vi "Control - Hybrid Engine.vi"() -> ()   [LabVIEW 2013]
uses:
  Control 2.ctl
  <vilib>/DAQmx/write.llb/DAQmx Write (Digital Bool 1Line 1Point).vi
  <vilib>/DAQmx/miscellaneous.llb/DAQmx Fill In Error Info.vi
panel:
  out "OFF":bool
  in  "Servo OFF Com":bool
  in  "Close Command":string="close!"
  in  "Open Command":string="open!"
  in  "Stop Button":bool
  in  "VISA resource name":refnum<visa-resource-name>="COM3"
  out "Servo Off":bool
  out "Servo On":bool
  in  "Serial Settings":T1={"baud rate"=9600, "data bits"=8, "parity"=enum."None", "stop bits"=10, "flow control"=0} {"flow control" items=["None"=0, "XON/XOFF"=1, "RTS/CTS"=2, "DTR/DSR"=4]; "stop bits" items=["1.0"=10, "1.5"=15, "2.0"=20]; "data bits" min=5 max=8 step=1; "baud rate" items=["75"=75, "110"=110, "134"=134, "150"=150, "300"=300, "600"=600, "1200"=1200, "1800"=1800, "2400"=2400, "4800"=4800, "7200"=7200, "9600"=9600, "14400"=14400, "19200"=19200, "28800"=28800, "38400"=38400, "56000"=56000, "57600"=57600, "115200"=115200, "128000"=128000, "230400"=230400]}
  in  "Servo ON Com":bool
  in  "Oxygen Flood":bool
  in  "Ignition":bool
  out "Disconnected":bool
  out "Solenoid \nClosed":bool
  out "Closed":bool
  out "READY":bool
  in  "Fill Line":bool
  out "FILL TANK EMPTYING":bool
  out "Venting":bool
  out "Filling":bool
  in  "Fill Line Vent":bool
  in  "Oxidizer Fill":bool
  # "***************THIS PROGRAM MUST BE RUNNING CONSTANTLY WHEN SOLENOIDS ARE CONNECTED"
  # "Engine Ignition"
  # "Oxidizer Filling"
  # "Manual Control"
  # "Must hold down to be activated"
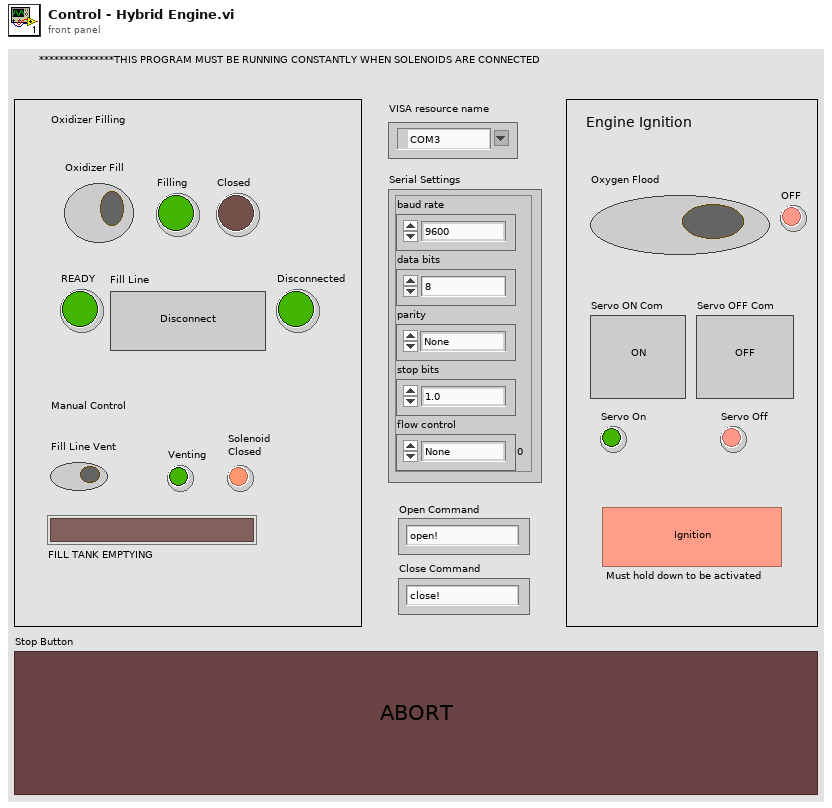
[diagram p1: front panel]
types:
  T1 = typedef "Control 2.ctl" = cluster{"baud rate":u32, "data bits":u16, "parity":enum16{"None", "Odd", "Even", "Mark", "Space"}, "stop bits":u16, "flow control":u16}
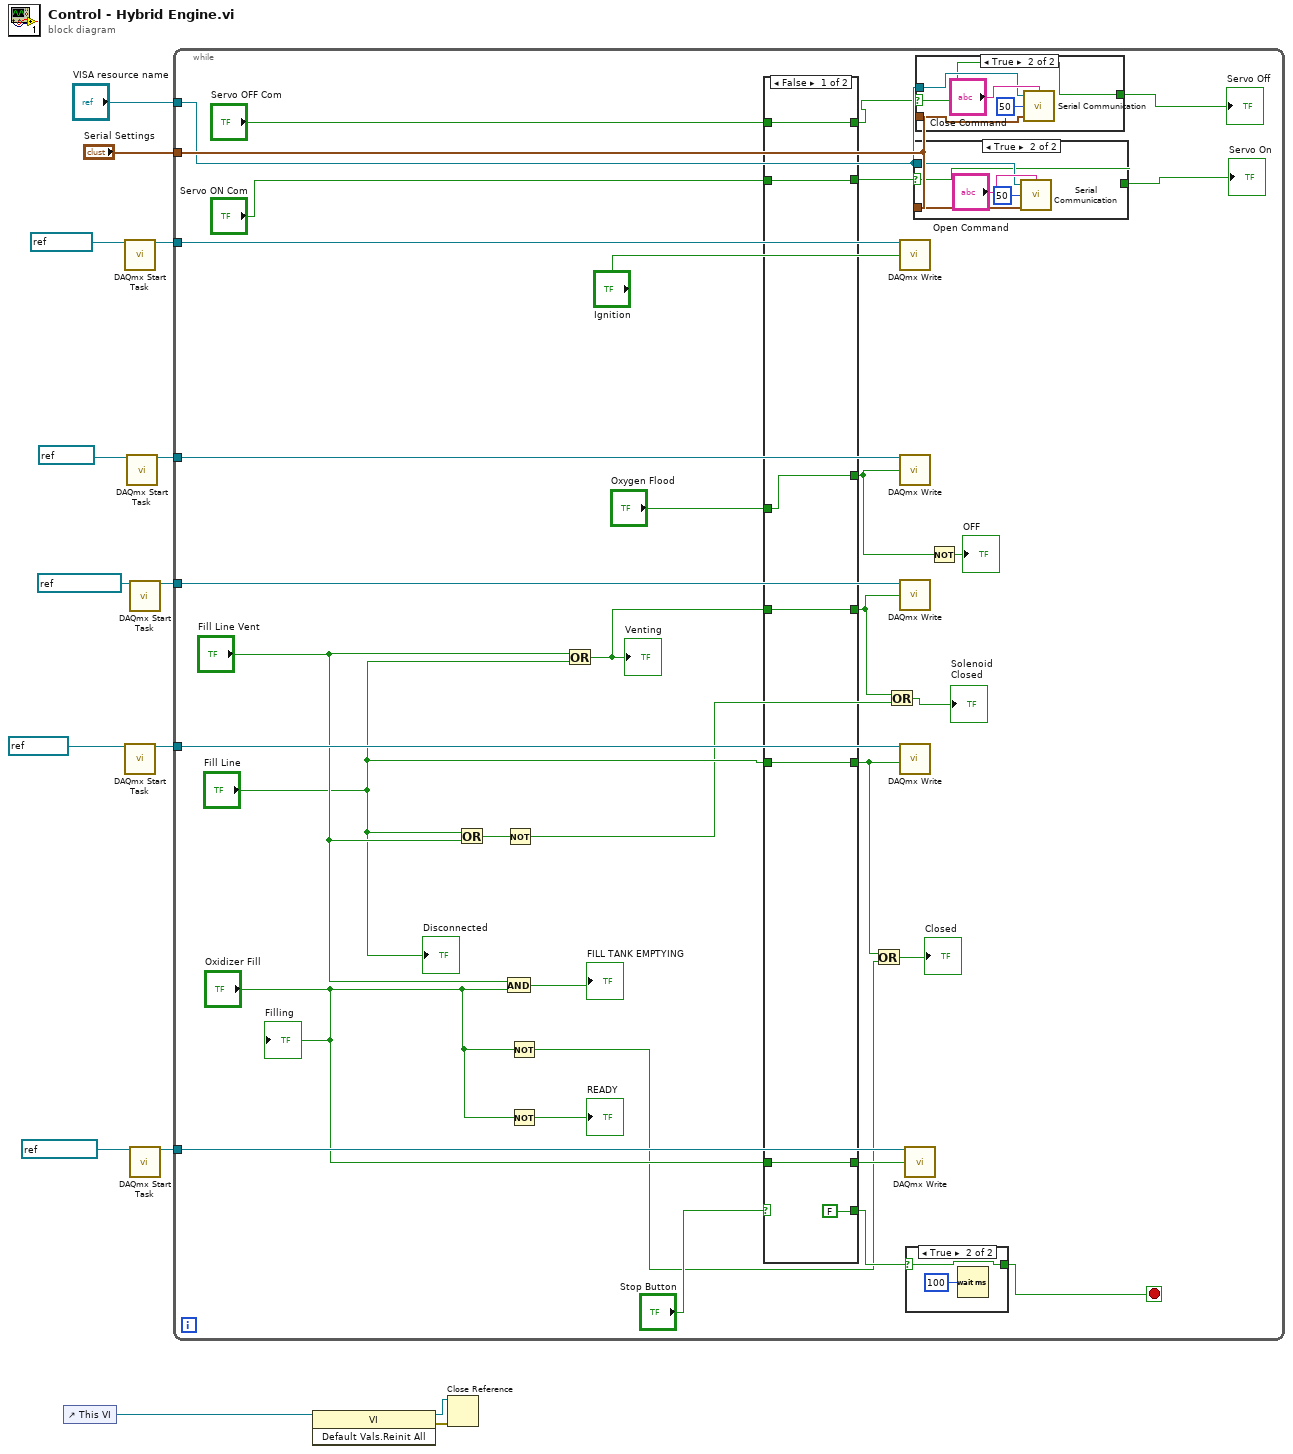
[diagram p0: block diagram]
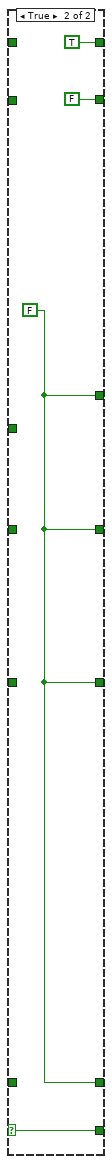
[diagram p3: hidden frame]
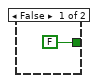
[diagram p4: hidden frame]
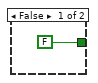
[diagram p5: hidden frame]
diagram:
  n1 = control-ref of="This VI"() -> (w1:refnum<vi>)
  n2 = call <vilib>:"DAQmx Start Task.vi"("task/channels in"=refnum<k21> "Igniter") -> ("task out"=w13:refnum<k21>)  [unwired: 13 in, 1 out]
  n3 = call <vilib>:"DAQmx Start Task.vi"("task/channels in"=refnum<k21> "AUX 1") -> ("task out"=w15:refnum<k21>)  [unwired: 13 in, 1 out]
  n4 = call <vilib>:"DAQmx Start Task.vi"("task/channels in"=refnum<k21> "O2fill") -> ("task out"=w6:refnum<k21>)  [unwired: 13 in, 1 out]
  n5 = call <vilib>:"DAQmx Start Task.vi"("task/channels in"=refnum<k21> "NOS VENT") -> ("task out"=w8:refnum<k21>)  [unwired: 13 in, 1 out]
  n6 = call <vilib>:"DAQmx Start Task.vi"("task/channels in"=refnum<k21> "NOS FILL") -> ("task out"=w14:refnum<k21>)  [unwired: 13 in, 1 out]
  n7 = while {
    tunnel: w15 -> [w49]
    tunnel: w14 -> [w48]
    tunnel: w13 -> [w47]
    tunnel: w8 -> [w46]
    tunnel: w6 -> [w44]
    tunnel: "VISA resource name" -> [w38]
    tunnel: "Serial Settings" -> [w39]
    stop <- w24 stop-if-true
    n8 = Or(x="Fill Line", y="Fill Line Vent") -> (x .or. y?=w42:bool)
    n9 = And(x="Fill Line Vent", y="Oxidizer Fill") -> (x .and. y?=→"FILL TANK EMPTYING":bool)
    n10 = Not(x=w42) -> (.not. x?=w20:bool)
    n11 = Not(x="Oxidizer Fill") -> (.not. x?=w23:bool)
    n12 = Not(x="Oxidizer Fill") -> (.not. x?=→"READY":bool)
    n13 = Or(x="Fill Line Vent", y="Fill Line") -> (x .or. y?=w30:bool)
    "Venting" <- w30
    n14 = case shown="False" "Stop Button" {
      selector: "Stop Button" -> [_ w60]
      tunnel: [w59 FALSE] -> w35
      tunnel: "Servo ON Com" -> [w59 _]
      tunnel: "Servo OFF Com" -> [w58 _]
      tunnel: [w58 TRUE] -> w32
      tunnel: "Oxygen Flood" -> [w57 _]
      tunnel: [w57 w63] -> w16
      tunnel: w30 -> [w56 _]
      tunnel: [w56 w63] -> w19
      tunnel: "Fill Line" -> [w55 _]
      tunnel: [w55 w63] -> w22
      tunnel: "Oxidizer Fill" -> [w54 _]
      tunnel: [w54 w63] -> w27
      tunnel: [FALSE w60] -> w25
      frame False {
      }
      frame True {
        w63 = FALSE
      }
    }
    n15 = Or(x=w22, y=w23) -> (x .or. y?=→"Closed":bool)
    n16 = Or(x=w19, y=w20) -> (x .or. y?=→"Solenoid \nClosed":bool)
    n17 = call-poly <vilib>:"DAQmx Write.vi"("task/channels in"=w47, "data"="Ignition") -> ()  [unwired: 11 in, 3 out]
    n18 = call-poly <vilib>:"DAQmx Write.vi"("task/channels in"=w44, "data"=w16) -> ()  [unwired: 11 in, 3 out]
    n19 = call-poly <vilib>:"DAQmx Write.vi"("task/channels in"=w46, "data"=w19) -> ()  [unwired: 11 in, 3 out]
    n20 = call-poly <vilib>:"DAQmx Write.vi"("task/channels in"=w49, "data"=w22) -> ()  [unwired: 11 in, 3 out]
    n21 = call-poly <vilib>:"DAQmx Write.vi"("task/channels in"=w48, "data"=w27) -> ()  [unwired: 11 in, 3 out]
    n22 = case shown="True" w25 {
      selector: w25 -> [w50 w51]
      tunnel: [w50 w51] -> w24
      frame False {
      }
      frame True {
        n23 = Wait (ms)(milliseconds to wait=u32 100) -> ()  [unwired: 1 out]
      }
    }
    n24 = case shown="True" w35 {
      selector: w35 -> [_ w65]
      tunnel: w39 -> [_ w68]
      tunnel: w38 -> [_ w67]
      tunnel: [FALSE w65] -> w36
      frame False {
      }
      frame True {
        n25 = call "Serial Communication.vi"("Command"="Open Command", "Serial Settings"=w68, "delay before read (ms)"=u32 50, "VISA resource name"=w67) -> ()  [unwired: 2 out]
      }
    }
    "Servo On" <- w36
    n26 = case shown="True" w32 {
      selector: w32 -> [_ w71]
      tunnel: w39 -> [_ w74]
      tunnel: w38 -> [_ w73]
      tunnel: [FALSE w71] -> w37
      frame False {
      }
      frame True {
        n27 = call "Serial Communication.vi"("Command"="Close Command", "Serial Settings"=w74, "delay before read (ms)"=u32 50, "VISA resource name"=w73) -> ()  [unwired: 2 out]
      }
    }
    "Servo Off" <- w37
    n28 = Not(x=w16) -> (.not. x?=→"OFF":bool)
    "Filling" <- "Oxidizer Fill"
    "Disconnected" <- "Fill Line"
  }
  n29 = invoke class="VI" method="Default Vals.Reinit All"(reference=w1) -> (reference out=w3:refnum<vi>, error out=w2:errorcluster)  [unwired: 2 in, 1 out]
  n30 = Close Reference(reference=w3, error in (no error)=w2) -> ()  [unwired: 1 out]
